vi "Rotate2Color.vi"() -> ()   [LabVIEW 2019]
uses:
  Placeholder_Colors.ctl
panel:
  out "Team_Desired":dbl
  in  "Colors Array":T1[](array[typedef])
  in  "Team_Current_Color":T1
  in  "Field_Desired":T1
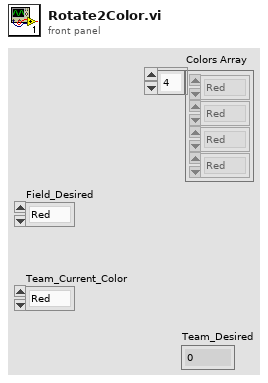
[diagram p1: front panel]
types:
  T1 = typedef "Placeholder_Colors.ctl" = enum16{"Red", "Yellow", "Blue", "Green"}
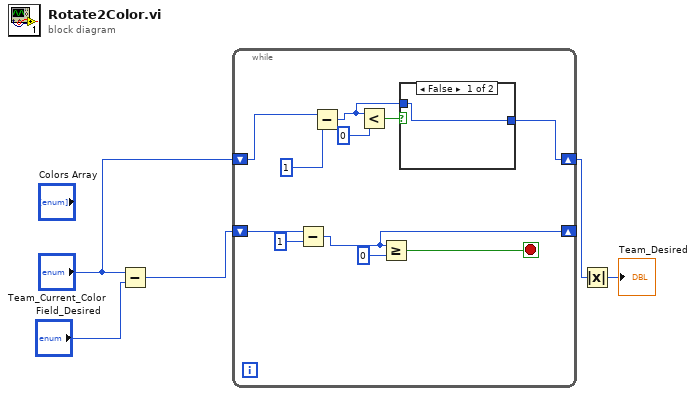
[diagram p0: block diagram]
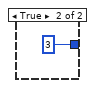
[diagram p2: hidden frame]
diagram:
  n1 = Subtract(x="Team_Current_Color", y="Field_Desired") -> (x-y=w3:u16)
  n2 = while {
    shift-right: [w6] -> _
    shift-left: w3 -> [w16]
    shift-right: [w8] -> w1
    shift-left: "Team_Current_Color" -> [w12]
    stop <- w13 stop-if-true
    n3 = Subtract(x=w16, y=u16 1) -> (x-y=w6:u16)
    n4 = Subtract(x=w12, y=1) -> (x-y=w7:i32)
    n5 = Less?(x=w7, y=0) -> (x < y?=w10:bool)
    n6 = Greater Or Equal?(x=w6, y=u16 0) -> (x >= y?=w13:bool)
    n7 = case shown="False" w10 {
      tunnel: [w17 3] -> w8
      tunnel: w7 -> [w17 _]
      frame False {
      }
      frame True {
      }
    }
  }
  n8 = Absolute Value(x=w1) -> (abs(x)=→"Team_Desired":i32)
